vi "Register Group.vi"(8 "error in (no error)":errorcluster, 10 "Group":refnum<class "GroupAbstract.lvclass">, 11 "Module in":refnum<class "Module.lvclass">) -> (0 "error out":errorcluster, 3 "Module out":refnum<class "Module.lvclass">)   [LabVIEW 2020, in "Volatus.lvlib" / "Module.lvclass"]
uses:
  Module.lvclass
  Module.lvclass/Module.ctl
  lv-vecto/Vecto/GroupAbstract/GroupAbstract.lvclass
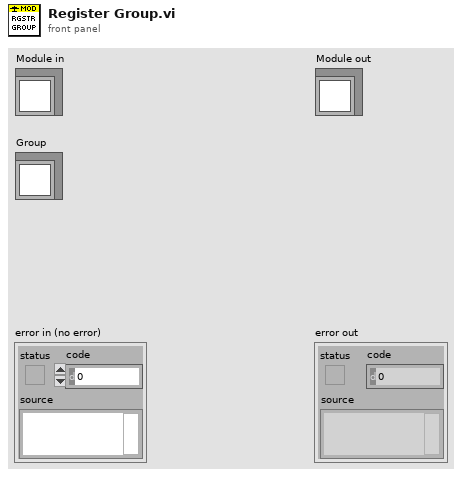
[diagram p1: front panel]
types:
  T1 = map{string, refnum<class "GroupAbstract.lvclass">}
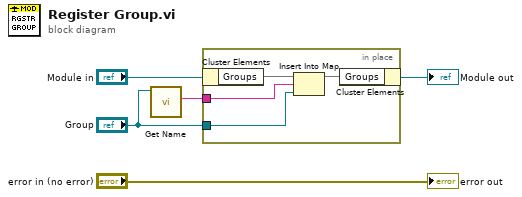
[diagram p0: block diagram]
diagram:
  n1 = call "Get Name.vi"("GroupAbstract in"="Group") -> ("Name"=w4:string)  [unwired: 8 in, 2 out]
  n2 = in-place {
    in-place-border: w4 -> [w8]
    in-place-border: "Group" -> [w7]
    n3 = in-place-cluster #1("Module in") -> ("Groups"=w9:T1)
    n4 = Insert Into Map(map in=w9, key=w8, value=w7) -> (map out=w6:T1)  [unwired: 2 out]
    n5 = in-place-cluster #1("Groups"=w6) -> (→"Module out":refnum<class "Module.lvclass">)
  }
  "error out" <- "error in (no error)"
